vi "Hash Core.vi"(6 "error in":errorcluster, 7 "Input String":string, 8 "s4 in":u32=271733878 format="%.0x", 9 "s3 in":u32=2562383102 format="%.0x", 10 "s2 in":u32=4023233417 format="%.0x", 11 "s1 in":u32=1732584193 format="%.0x") -> (0 "s4 out":u32, 1 "s3 out":u32, 2 "s2 out":u32, 3 "s1 out":u32, 4 "error out":errorcluster)   [LabVIEW 2022 SP3, in "hse-misc.lvlib"]
doc: "____\nHAMPEL SOFTWARE ENGINEERING v3.8.0 (2023-12-18 14:41)"
uses:
  hse-misc.lvlib
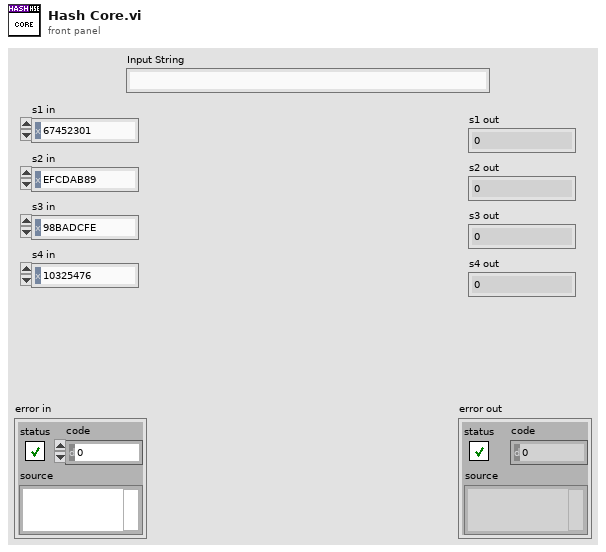
[diagram p1: front panel]
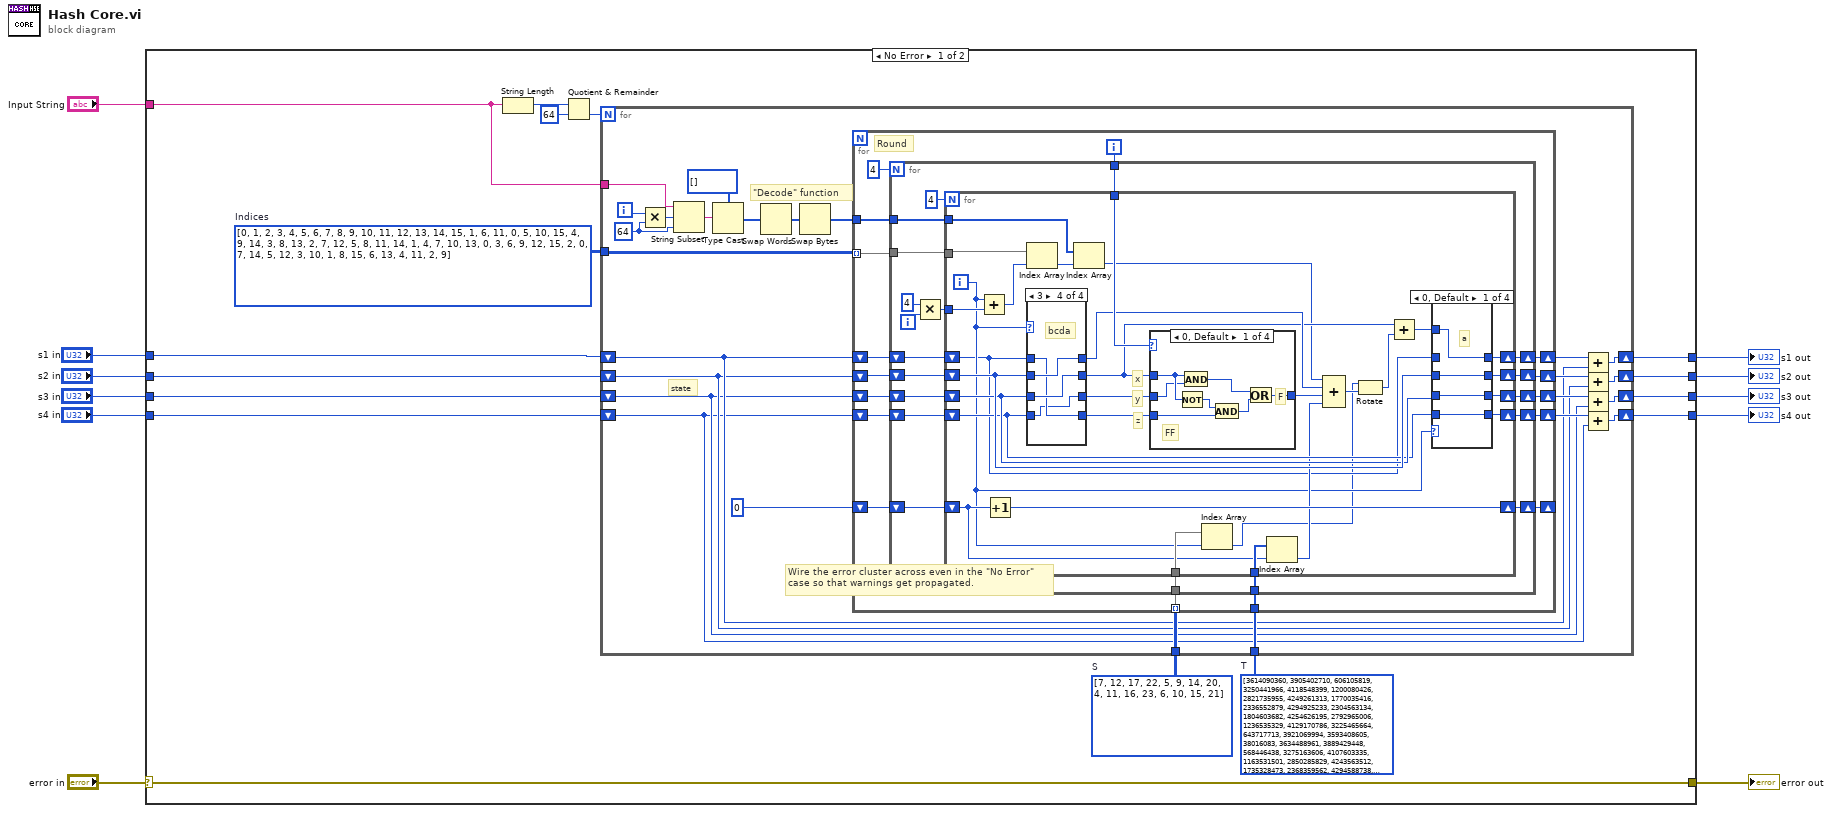
[diagram p0: block diagram]
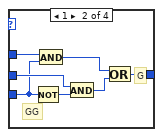
[diagram p2: hidden frame]
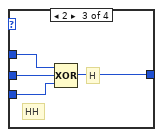
[diagram p3: hidden frame]
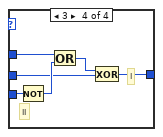
[diagram p4: hidden frame]
diagram:
  n1 = case shown="No Error" "error in" {
    selector: "error in" -> [w27 w174]
    tunnel: [w27 w174] -> w10
    tunnel: [w20 _] -> w9
    tunnel: [w19 _] -> w8
    tunnel: [w18 _] -> w7
    tunnel: [w17 _] -> w6
    tunnel: "Input String" -> [w16 _]
    tunnel: "s1 in" -> [w15 _]
    tunnel: "s2 in" -> [w14 _]
    tunnel: "s3 in" -> [w13 _]
    tunnel: "s4 in" -> [w12 _]
    frame No Error {
      w21 = i32[][] [[7, 12, 17, 22], [5, 9, 14, 20], [4, 11, 16, 23], [6, 10, 15, 21]]  # S
      w22 = u32[] [3614090360, 3905402710, 606105819, 3250441966, 4118548399, 1200080426, 2821735955, 4249261313, 1770035416, 2336552879, 4294925233, 2304563134, 1804603682, 4254626195, 2792965006, 1236535329, 4129170786, 3225465664, 643717713, 3921069994, 3593408605, 38016083, 3634488961, 3889429448, 568446438, 3275163606, 4107603335, 1163531501, 2850285829, 4243563512, 1735328473, 2368359562, 4294588738, 2272392833, 1839030562, 4259657740, 2763975236, 1272893353, 4139469664, 3200236656, 681279174, 3936430074, 3572445317, 76029189, 3654602809, 3873151461, 530742520, 3299628645, 4096336452, 1126891415, 2878612391, 4237533241, 1700485571, 2399980690, 4293915773, 2240044497, 1873313359, 4264355552, 2734768916, 1309151649, 4149444226, 3174756917, 718787259, 3951481745]  # T
      w23 = i32[][] [[0, 1, 2, 3, 4, 5, 6, 7, 8, 9, 10, 11, 12, 13, 14, 15], [1, 6, 11, 0, 5, 10, 15, 4, 9, 14, 3, 8, 13, 2, 7, 12], [5, 8, 11, 14, 1, 4, 7, 10, 13, 0, 3, 6, 9, 12, 15, 2], [0, 7, 14, 5, 12, 3, 10, 1, 8, 15, 6, 13, 4, 11, 2, 9]]  # Indices
      # "Wire the error cluster across even in the \"No Error\"\ncase so that warnings get propagated."
      n2 = String Length(string=w16) -> (length=w25:i32)
      n3 = Quotient & Remainder(x=w25, y=64) -> (floor(x/y)=w26:i32)  [unwired: 1 out]
      n4 = for {
        N: w26 -> [_]
        tunnel: w23 -> [w47]
        tunnel: w22 -> [w46]
        tunnel: w21 -> [w45]
        shift-right: [w44] -> w20
        shift-left: w15 -> [w40]
        shift-right: [w43] -> w19
        shift-left: w14 -> [w39]
        shift-right: [w42] -> w18
        shift-left: w13 -> [w38]
        shift-right: [w41] -> w17
        shift-left: w12 -> [w37]
        tunnel: w16 -> [w35]
        i -> [w36]
        w31 = 64 ("y")
        # "\"Decode\" function"
        # "state"
        n5 = Multiply(x=w36, y=w31) -> (x*y=w32:i32)
        n6 = String Subset(string=w35, offset (0)=w32, length (rest)=w31) -> (substring=w34:string)
        n7 = Type Cast(type=u32[] [], x=w34) -> (*(type *) &x=w29:u32[])
        n8 = Swap Words(1:w29) -> (0:w30:u32[])
        n9 = Swap Bytes(anything=w30) -> (byte swapped=w28:u32[])
        n10 = for {
          shift-right: [w63] -> w49
          shift-left: w40 -> [w64]
          shift-right: [w62] -> w50
          shift-left: w39 -> [w65]
          shift-right: [w61] -> w51
          shift-left: w38 -> [w66]
          shift-right: [w60] -> w52
          shift-left: w37 -> [w67]
          tunnel: w47 -> [w59] mode=indexing
          tunnel: w45 -> [w58] mode=indexing
          tunnel: w28 -> [w57]
          shift-right: [w54] -> _
          shift-left: 0 -> [w55]
          tunnel: w46 -> [w53]
          i -> [w68]
          # "Round"
          n11 = for {
            N: 4 -> [_]
            tunnel: w68 -> [w87]
            shift-right: [w80] -> w60
            shift-left: w67 -> [w81]
            shift-right: [w79] -> w61
            shift-left: w66 -> [w82]
            shift-right: [w85] -> w62
            shift-left: w65 -> [w83]
            shift-right: [w86] -> w63
            shift-left: w64 -> [w84]
            tunnel: w59 -> [w78]
            tunnel: w58 -> [w77]
            tunnel: w57 -> [w73]
            shift-right: [w70] -> w54
            shift-left: w55 -> [w71]
            tunnel: w53 -> [w69]
            i -> [w76]
            n12 = Multiply(x=4, y=w76) -> (x*y=w74:i32)
            n13 = for {
              N: 4 -> [_]
              tunnel: w87 -> [w99]
              shift-right: [w109] -> w80
              shift-left: w81 -> [w104]
              shift-right: [w108] -> w79
              shift-left: w82 -> [w105]
              shift-right: [w107] -> w85
              shift-left: w83 -> [w106]
              shift-right: [w110] -> w86
              shift-left: w84 -> [w90]
              tunnel: w78 -> [w117]
              tunnel: w77 -> [w116]
              tunnel: w74 -> [w103]
              tunnel: w73 -> [w113]
              shift-right: [w100] -> w70
              shift-left: w71 -> [w101]
              tunnel: w69 -> [w102]
              i -> [w91]
              # "z"
              # "y"
              # "x"
              n14 = Add(x=w91, y=w103) -> (x+y=w115:i32)
              n15 = Increment(x=w101) -> (x+1=w100:i32)
              n16 = Index Array(array=w117, index=w115) -> (element=w114:i32)
              n17 = case shown="3" w91 {
                tunnel: w90 -> [w161 w164 w167 w171]
                tunnel: w106 -> [w160 w163 w166 w173]
                tunnel: w105 -> [w159 w162 w169 w172]
                tunnel: w104 -> [w158 w165 w168 w170]
                tunnel: [w161 w165 w169 w173] -> w94
                tunnel: [w160 w164 w168 w172] -> w93
                tunnel: [w159 w163 w167 w170] -> w112
                tunnel: [w158 w162 w166 w171] -> w111
                frame 0, Default {
                  # "abcd"
                }
                frame 1 {
                  # "dabc"
                }
                frame 2 {
                  # "cdab"
                }
                frame 3 {
                  # "bcda"
                }
              }
              n18 = Index Array(array=w113, index=w114) -> (element=w88:u32)
              n19 = case shown="0, Default" w99 {
                tunnel: w93 -> [w121 w127 w134 w138]
                tunnel: w112 -> [w120 w126 w135 w137]
                tunnel: w111 -> [w119 w125 w133 w136]
                tunnel: [w118 w128 w132 w139] -> w95
                frame 0, Default {
                  # "FF"
                  # "F"
                  n20 = Not(x=w121) -> (.not. x?=w124:u32)
                  n21 = And(x=w121, y=w120) -> (x .and. y?=w123:u32)
                  n22 = And(x=w124, y=w119) -> (x .and. y?=w122:u32)
                  n23 = Or(x=w123, y=w122) -> (x .or. y?=w118:u32)
                }
                frame 1 {
                  # "GG"
                  # "G"
                  n24 = Not(x=w125) -> (.not. x?=w129:u32)
                  n25 = And(x=w127, y=w125) -> (x .and. y?=w130:u32)
                  n26 = And(x=w126, y=w129) -> (x .and. y?=w131:u32)
                  n27 = Or(x=w130, y=w131) -> (x .or. y?=w128:u32)
                }
                frame 2 {
                  # "H"
                  # "HH"
                  n28 = Compound Arithmetic op=XOR(w134, w135, w133) -> (w132:u32)
                }
                frame 3 {
                  # "I"
                  # "II"
                  n29 = Not(x=w136) -> (.not. x?=w141:u32)
                  n30 = Or(x=w138, y=w141) -> (x .or. y?=w140:u32)
                  n31 = Exclusive Or(1:w137, 2:w140) -> (0:w139:u32)
                }
              }
              n32 = Index Array(array=w116, index=w91) -> (element=w89:i32)
              n33 = Index Array(array=w102, index=w101) -> (element=w96:u32)
              n34 = Compound Arithmetic op=ADD(w88, w94, w95, w96) -> (w98:u32)
              n35 = Rotate(1:w98, 2:w89) -> (0:w92:u32)
              n36 = Add(x=w93, y=w92) -> (x+y=w97:u32)
              n37 = case shown="0, Default" w91 {
                tunnel: w97 -> [w145 w149 w153 w157]
                tunnel: [w145 w148 w152 w156] -> w110
                tunnel: [w142 w149 w150 w154] -> w109
                tunnel: [w143 w146 w153 w155] -> w108
                tunnel: [w144 w147 w151 w157] -> w107
                tunnel: w90 -> [_ w148 w152 w156]
                tunnel: w106 -> [w144 w147 w151 _]
                tunnel: w105 -> [w143 w146 _ w155]
                tunnel: w104 -> [w142 _ w150 w154]
                frame 0, Default {
                  # "a"
                }
                frame 1 {
                  # "d"
                }
                frame 2 {
                  # "c"
                }
                frame 3 {
                  # "b"
                }
              }
            }
          }
        }
        n38 = Add(x=w49, y=w40) -> (x+y=w44:u32)
        n39 = Add(x=w50, y=w39) -> (x+y=w43:u32)
        n40 = Add(x=w51, y=w38) -> (x+y=w42:u32)
        n41 = Add(x=w52, y=w37) -> (x+y=w41:u32)
      }
    }
    frame Error {
    }
  }
  "error out" <- w10
  "s1 out" <- w9
  "s2 out" <- w8
  "s3 out" <- w7
  "s4 out" <- w6
